vi "Home Stage.vi"(7 "Direction":enum16{"- infinity", "+ infinity"}(ring)=enum."+ infinity", 8 "error in (no error)":errorcluster, 9 "Timeout (sec)":dbl=100.0, 10 "Index":i32, 11 "Visa Array in":refnum<visa-resource-name>[](array[refnum])) -> (0 "error out":errorcluster, 1 "Time out":bool, 3 "Visa Array out":refnum<visa-resource-name>[](array[refnum]))   [LabVIEW 2010, in "SignalWriterMH110203USBStepperMotor.lvclass"]
uses:
  SignalWriterMH110203USBStepperMotor.lvclass
  class_data.vi
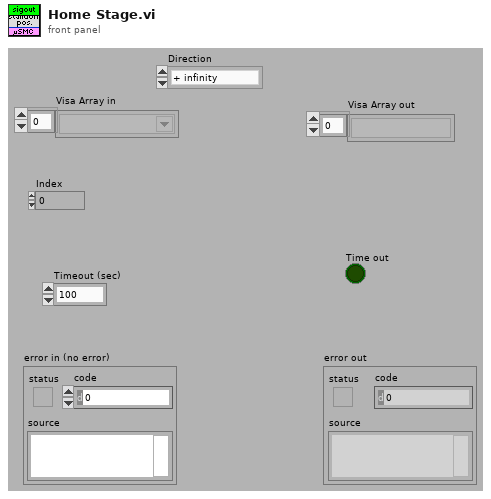
[diagram p1: front panel]
types:
  T1 = typedef "SignalWriterMH110203USBStepperMotor.lvclass/GoTo Control (uSMC).ctl" = cluster{"Step motor ID":string, "SMname":string, "Backlash":u16, "wait for input sygnal to start":bool, "use slow start/stop":bool, "units name":string, "Maximum speed":dbl, "speed":dbl, "step":u8, "point 1 ticks":i32, "point 2 ticks":i32, "point 1 units":dbl, "point 2 units":dbl, "Limit Switch standoff":dbl, "Zero Value":dbl, "Destination Position":dbl, "force backlash":bool, "power off when stop":bool, "POff delay":dbl, "positioner name":string, "R, Ohm":dbl, "I, mA":dbl, "Positioner's Type":u16, "Reset Direction":bool, "Manufacturer":string, "Model":string, "Scheme":string, "FirmwareVer":string}
  T2 = typedef "SignalWriterMH110203USBStepperMotor.lvclass/Get State Control (uSMC).ctl" = cluster{"Current Posistion":dbl, "CW/CCW":bool, "Speed":u16, "Temperature":dbl, "Power":u16, "Limit Switch 1":bool, "Limit Switch 2":bool, "After Reset":bool, "Step":u8, "Backlash":bool, "RT Error":bool, "RT State":bool, "Sync In":bool, "Sync Out":bool, "Ext Disconnect":bool, "Usb Powered":bool, "Voltage":dbl, "Working":bool, "SM Position in Encoder Units":i32, "Encoder Current Position":i32}
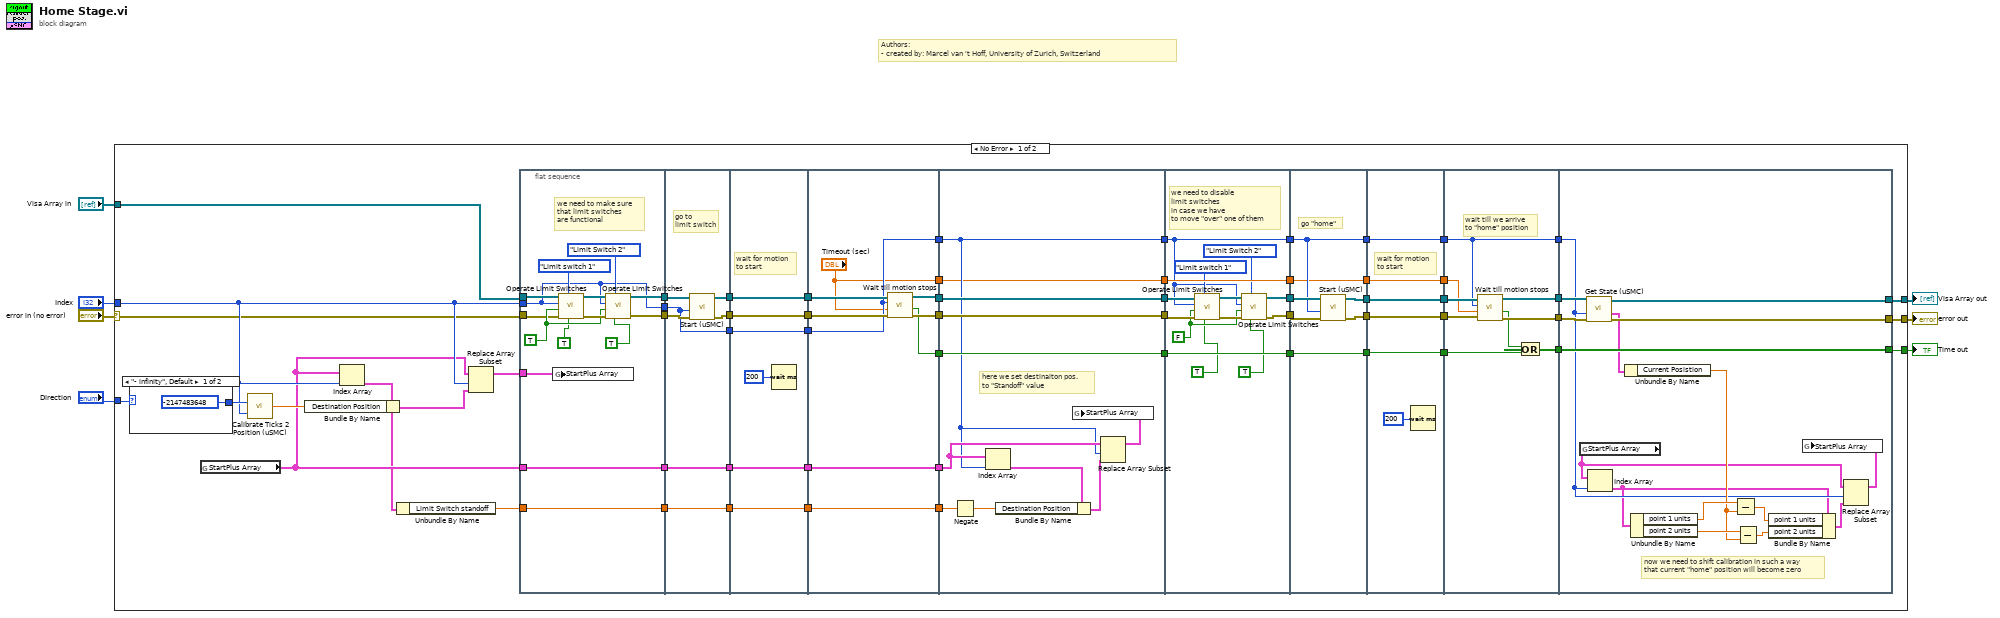
[diagram p0: block diagram]
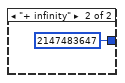
[diagram p2: hidden frame]
diagram:
  # "Authors: \n- created by: Marcel van 't Hoff, University of Zurich, Switzerland"
  n1 = case shown="No Error" "error in (no error)" {
    selector: "error in (no error)" -> [w8 w171]
    tunnel: "Direction" -> [w20 _]
    tunnel: "Index" -> [w16 _]
    tunnel: "Visa Array in" -> [w14 w170]
    tunnel: [w11 w170] -> w4
    tunnel: [w10 w171] -> w1
    tunnel: [w9 _] -> w3
    frame No Error {
      n2 = case shown="\"- infinity\", Default" w20 {
        tunnel: [-2147483648 ("ticks") 2147483647 ("ticks")] -> w19
        frame "- infinity", Default {
        }
        frame "+ infinity" {
        }
      }
      n3 = global read "class_data.vi" "StartPlus Array"() -> (w15:T1[])
      n4 = call "Calibrate Ticks 2 Position (uSMC).vi"("array index"=w16, "ticks"=w19) -> ("value"=w18:dbl)
      n5 = Index Array(array=w15, index=w16) -> (element=w13:T1)
      n6 = Bundle By Name(cluster=w13, "Destination Position"=w18) -> (w17:T1)
      n7 = Unbundle By Name(w13) -> ("Limit Switch standoff"=w12:dbl)
      n8 = Replace Array Subset(array=w15, new element=w17, index=w16) -> (w21:T1[])
      n9 = flat-sequence {
        tunnel: w16 -> [w72]
        tunnel: w8 -> [w73]
        tunnel: w14 -> [w77]
        tunnel: [w76] -> w67
        tunnel: [w72] -> w65
        tunnel: w21 -> [w84]
        tunnel: [w83] -> w64
        tunnel: w15 -> [w83]
        tunnel: [w82] -> w63
        tunnel: w12 -> [w82]
        tunnel: [w75] -> w66
        tunnel: w67 -> [w91]
        tunnel: w66 -> [w89]
        tunnel: w65 -> [w87]
        tunnel: [w90] -> w62
        tunnel: [w88] -> w61
        tunnel: [w87] -> w60
        tunnel: [w86] -> w59
        tunnel: w64 -> [w86]
        tunnel: [w85] -> w58
        tunnel: w63 -> [w85]
        tunnel: w62 -> [w97]
        tunnel: w61 -> [w96]
        tunnel: w60 -> [w95]
        tunnel: [w97] -> w57
        tunnel: [w96] -> w56
        tunnel: [w95] -> w55
        tunnel: [w93] -> w54
        tunnel: w59 -> [w93]
        tunnel: [w92] -> w53
        tunnel: w58 -> [w92]
        tunnel: w57 -> [w106]
        tunnel: w56 -> [w105]
        tunnel: w55 -> [w100]
        tunnel: [w104] -> w52
        tunnel: [w103] -> w51
        tunnel: [w102] -> w50
        tunnel: w54 -> [w102]
        tunnel: [w101] -> w49
        tunnel: w53 -> [w101]
        tunnel: [w100] -> w48
        tunnel: [w98] -> w47
        tunnel: ["Timeout (sec)"] -> w46
        tunnel: w52 -> [w117]
        tunnel: w51 -> [w116]
        tunnel: w50 -> [w111]
        tunnel: w49 -> [w112]
        tunnel: [w117] -> w45
        tunnel: [w116] -> w44
        tunnel: [w110] -> w43
        tunnel: w48 -> [w110]
        tunnel: [w115] -> w42
        tunnel: w47 -> [w115]
        tunnel: [w108] -> w41
        tunnel: w46 -> [w108]
        tunnel: w45 -> [w129]
        tunnel: [w127] -> w40
        tunnel: w44 -> [w125]
        tunnel: w43 -> [w121]
        tunnel: [w121] -> w38
        tunnel: w42 -> [w131]
        tunnel: [w131] -> w37
        tunnel: w41 -> [w130]
        tunnel: [w130] -> w36
        tunnel: [w126] -> w39
        tunnel: w40 -> [w138]
        tunnel: w39 -> [w137]
        tunnel: w38 -> [w133]
        tunnel: w37 -> [w134]
        tunnel: [w136] -> w35
        tunnel: [w135] -> w34
        tunnel: [w134] -> w33
        tunnel: [w133] -> w32
        tunnel: [w132] -> w31
        tunnel: w36 -> [w132]
        tunnel: w35 -> [w144]
        tunnel: [w144] -> w30
        tunnel: w34 -> [w143]
        tunnel: [w143] -> w29
        tunnel: w33 -> [w142]
        tunnel: [w142] -> w28
        tunnel: w32 -> [w141]
        tunnel: [w141] -> w27
        tunnel: w31 -> [w140]
        tunnel: [w140] -> w26
        tunnel: w30 -> [w153]
        tunnel: w29 -> [w152]
        tunnel: w28 -> [w148]
        tunnel: w27 -> [w146]
        tunnel: w26 -> [w151]
        tunnel: [w150] -> w25
        tunnel: [w149] -> w24
        tunnel: [w147] -> w23
        tunnel: [w146] -> w22
        tunnel: [w169] -> w9
        tunnel: [w165] -> w10
        tunnel: [w166] -> w11
        tunnel: w25 -> [w167]
        tunnel: w24 -> [w168]
        tunnel: w23 -> [w169]
        tunnel: w22 -> [w157]
        frame #0 {
          w74 = TRUE ("Use switch?")
          # "we need to make sure\nthat limit switches\nare functional"
          n10 = global write "class_data.vi" "StartPlus Array"(w84) -> ()
          n11 = call "Operate Limit Switches.vi"("True state"=TRUE ("Use switch?"), "Limit switch selector"=enum16{"Limit switch 1", "Limit Switch 2"}."Limit switch 1", "error in (no error)"=w73, "Use switch?"=w74, "Index"=w72, "Visa Array in"=w77) -> ("error out"=w79:errorcluster, "Visa Array out"=w78:refnum<visa-resource-name>[])  [unwired: 4 in]
          n12 = call "Operate Limit Switches.vi"("True state"=TRUE ("Use switch?"), "Limit switch selector"=enum16{"Limit switch 1", "Limit Switch 2"}."Limit Switch 2", "error in (no error)"=w79, "Use switch?"=w74, "Index"=w72, "Visa Array in"=w78) -> ("error out"=w75:errorcluster, "Visa Array out"=w76:refnum<visa-resource-name>[])  [unwired: 4 in]
        }
        frame #1 {
          # "go to\nlimit switch"
          n13 = call "Start (uSMC).vi"("error in"=w89, "Index"=w87, "Visa Array In"=w91) -> ("error out"=w88:errorcluster, "Visa Array Out"=w90:refnum<visa-resource-name>[])  [unwired: 7 in]
        }
        frame #2 {
          # "wait for motion\nto start"
          n14 = Wait (ms)(milliseconds to wait=u32 200) -> ()  [unwired: 1 out]
        }
        frame #3 {
          n15 = call "Wait till motion stops.vi"("error in"=w105, "Timeout (sec)"="Timeout (sec)", "Index"=w100, "Visa Array Out"=w106) -> ("error out"=w103:errorcluster, "Time out?"=w98:bool, "Visa array out"=w104:refnum<visa-resource-name>[])  [unwired: 4 in, 1 out]
        }
        frame #4 {
          # "here we set destinaiton pos.\nto \"Standoff\" value"
          n16 = Negate(x=w112) -> (-x=w109:dbl)
          n17 = Index Array(array=w111, index=w110) -> (element=w107:T1)
          n18 = Bundle By Name(cluster=w107, "Destination Position"=w109) -> (w114:T1)
          n19 = Replace Array Subset(array=w111, new element=w114, index=w110) -> (w113:T1[])
          n20 = global write "class_data.vi" "StartPlus Array"(w113) -> ()
        }
        frame #5 {
          w120 = FALSE ("Use switch?")
          # "we need to disable\nlimit switches\nin case we have\nto move \"over\" one of them"
          n21 = call "Operate Limit Switches.vi"("True state"=TRUE ("Use switch?"), "Limit switch selector"=enum16{"Limit switch 1", "Limit Switch 2"}."Limit switch 1", "error in (no error)"=w125, "Use switch?"=w120, "Index"=w121, "Visa Array in"=w129) -> ("error out"=w124:errorcluster, "Visa Array out"=w128:refnum<visa-resource-name>[])  [unwired: 4 in]
          n22 = call "Operate Limit Switches.vi"("True state"=TRUE ("Use switch?"), "Limit switch selector"=enum16{"Limit switch 1", "Limit Switch 2"}."Limit Switch 2", "error in (no error)"=w124, "Use switch?"=w120, "Index"=w121, "Visa Array in"=w128) -> ("error out"=w126:errorcluster, "Visa Array out"=w127:refnum<visa-resource-name>[])  [unwired: 4 in]
        }
        frame #6 {
          # "go \"home\""
          n23 = call "Start (uSMC).vi"("error in"=w137, "Index"=w133, "Visa Array In"=w138) -> ("error out"=w135:errorcluster, "Visa Array Out"=w136:refnum<visa-resource-name>[])  [unwired: 7 in]
        }
        frame #7 {
          # "wait for motion\nto start"
          n24 = Wait (ms)(milliseconds to wait=u32 200) -> ()  [unwired: 1 out]
        }
        frame #8 {
          # "wait till we arrive\nto \"home\" position"
          n25 = call "Wait till motion stops.vi"("error in"=w152, "Timeout (sec)"=w151, "Index"=w146, "Visa Array Out"=w153) -> ("error out"=w149:errorcluster, "Time out?"=w145:bool, "Visa array out"=w150:refnum<visa-resource-name>[])  [unwired: 4 in, 1 out]
          n26 = Or(x=w145, y=w148) -> (x .or. y?=w147:bool)
        }
        frame #9 {
          # "now we need to shift calibration in such a way\nthat current \"home\" position will become zero"
          n27 = global read "class_data.vi" "StartPlus Array"() -> (w158:T1[])
          n28 = call "Get State (uSMC).vi"("error in (no error)"=w168, "SM number"=w157, "Visa array in"=w167) -> ("error out"=w165:errorcluster, "State cluster"=w164:T2, "Visa array out"=w166:refnum<visa-resource-name>[])  [unwired: 6 in]
          n29 = Index Array(array=w158, index=w157) -> (element=w155:T1)
          n30 = Unbundle By Name(w164) -> ("Current Posistion"=w161:dbl)
          n31 = Unbundle By Name(w155) -> ("point 1 units"=w163:dbl, "point 2 units"=w162:dbl)
          n32 = Subtract(x=w163, y=w161) -> (x-y=w160:dbl)
          n33 = Subtract(x=w162, y=w161) -> (x-y=w159:dbl)
          n34 = Bundle By Name(cluster=w155, "point 1 units"=w160, "point 2 units"=w159) -> (w156:T1)
          n35 = Replace Array Subset(array=w158, new element=w156, index=w157) -> (w154:T1[])
          n36 = global write "class_data.vi" "StartPlus Array"(w154) -> ()
        }
      }
    }
    frame Error {
    }
  }
  "Visa Array out" <- w4
  "error out" <- w1
  "Time out" <- w3
